vi "CloseExcel.vi"(8 "错误输入（无错误）":errorcluster, 11 "Open":refnum<k7>) -> (0 "错误输出":errorcluster)   [LabVIEW 2017]
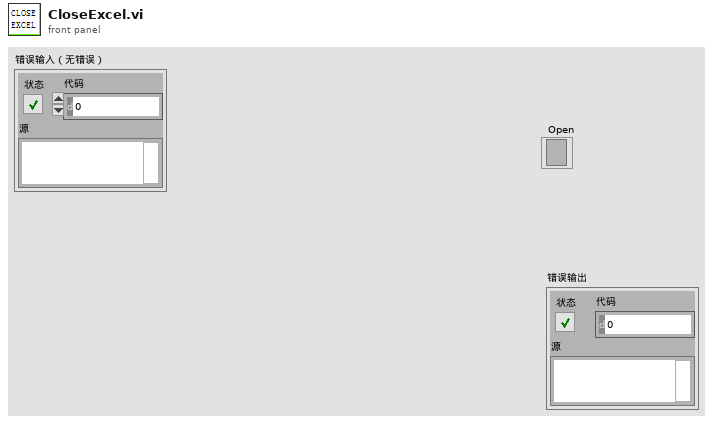
[diagram p1: front panel]
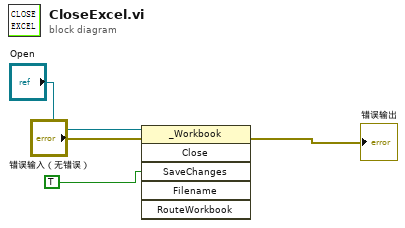
[diagram p0: block diagram]
diagram:
  n1 = invoke on="调用节点" class="_Workbook" method="Close"(reference="Open", error in="错误输入（无错误）", "SaveChanges"=TRUE ("布尔")) -> (error out=→"错误输出":errorcluster)  [unwired: 3 in, 5 out]
